vi "calculate stack progress.vi"(8 "error in (no error)":errorcluster, 11 "Autofocus in":refnum<class "Autofocus.lvclass">) -> (0 "error out":errorcluster, 3 "Autofocus out":refnum<class "Autofocus.lvclass">)   [LabVIEW 2012, in "Autofocus.lvclass"]
uses:
  Autofocus.lvclass
  Autofocus.lvclass/Autofocus.ctl
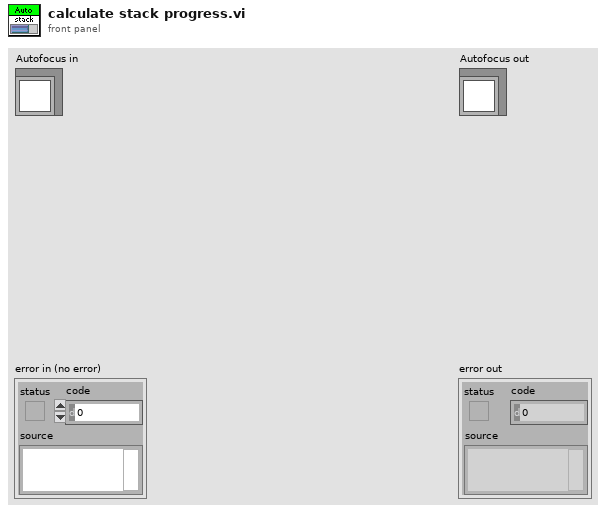
[diagram p1: front panel]
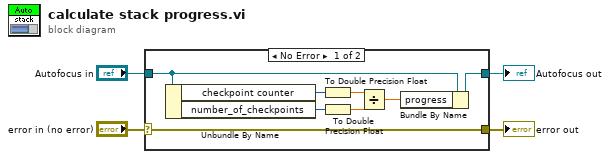
[diagram p0: block diagram]
diagram:
  n1 = case shown="No Error" "error in (no error)" {
    selector: "error in (no error)" -> [w12 w14]
    tunnel: [w12 w14] -> w3
    tunnel: [w6 w13] -> w1
    tunnel: "Autofocus in" -> [w7 w13]
    frame No Error {
      n2 = Unbundle By Name(w7) -> ("checkpoint counter"=w11:i32, "number_of_checkpoints"=w10:u16)
      n3 = To Double Precision Float(number=w11) -> (double precision float=w9:dbl)
      n4 = To Double Precision Float(number=w10) -> (double precision float=w8:dbl)
      n5 = Divide(x=w9, y=w8) -> (x/y=w5:dbl)
      n6 = Bundle By Name(cluster=w7, "progress"=w5) -> (w6:refnum<class "Autofocus.lvclass">)
    }
    frame Error {
    }
  }
  "error out" <- w3
  "Autofocus out" <- w1
